vi "Set Sensor Mode.vi"(8 "error in (no error)":errorcluster, 10 "Sensor Mode":T1(ring), 11 "FW102C in":i32) -> (0 "error out":errorcluster, 3 "FW102C out":i32)   [LabVIEW 2018, in "Thorlabs_FW102C.lvlib"]
doc: "sensors=0 Sensors turn off when wheel is idle to eliminate stray light\nsensors=1 Sensors remain active"
uses:
  Thorlabs_FW102C.lvlib
  <instrlib>/Thorlabs_FW102C/Library/FilterWheel102_win32.dll
  Library/FilterWheel102_win64.dll
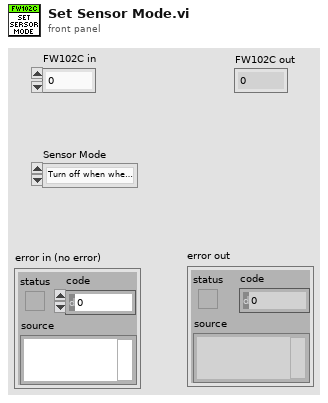
[diagram p1: front panel]
types:
  T1 = enum16{"Turn off when wheel is idle to eliminate stray light", "Remain active"}
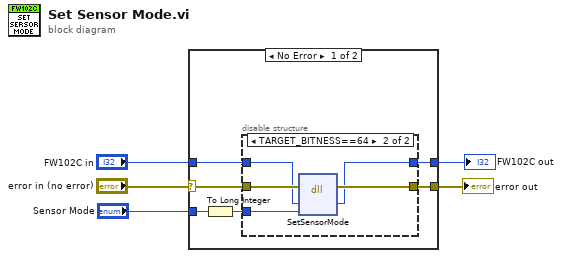
[diagram p0: block diagram]
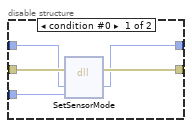
[diagram p2: hidden frame]
diagram:
  n1 = case shown="No Error" "error in (no error)" {
    selector: "error in (no error)" -> [w11 w22]
    tunnel: [w10 w22] -> w5
    tunnel: "FW102C in" -> [w9 w23]
    tunnel: [w8 w23] -> w2
    tunnel: "Sensor Mode" -> [w7 _]
    frame No Error {
      n2 = To Long Integer(number=w7) -> (32bit integer=w6:i32)
      n3 = disable-structure shown="TARGET_BITNESS==64" {
        disable-tunnel: w11 -> [w16 w21]
        disable-tunnel: [w15 w20] -> w10
        disable-tunnel: w9 -> [w14 w19]
        disable-tunnel: [w13 w18] -> w8
        disable-tunnel: w6 -> [w12 w17]
        frame condition #0 {
          n4 = dll-call lib="E:/Program Files (x86)/National Instruments/LabVIEW 2011/instr.lib/Thorlabs_FW102C/Library/FilterWheel102_win32.dll" fn="SetSensorMode"(error in=w16, "hdl"=w14, "sensor mode"=w12) -> (error out=w15:errorcluster, "hdl"=w13:i32)  [unwired: 4 in, 1 out]
        }
        frame condition #1 (active) {
          n5 = dll-call lib="C:/Users/astrolab/Desktop/Labview_code/Thorlabs_FW102C/Library/FilterWheel102_win64.dll" fn="SetSensorMode"(error in=w21, "hdl"=w19, "sensor mode"=w17) -> (error out=w20:errorcluster, "hdl"=w18:i32)  [unwired: 4 in, 1 out]
        }
      }
    }
    frame Error {
    }
  }
  "error out" <- w5
  "FW102C out" <- w2
